vi "setSetpoints.vi"(0 "Interface in":T2, 5 "Setpoint":T1, 7 "Value":sgl, 11 "error in":errorcluster) -> (4 "Interface out":T2, 15 "error out":errorcluster)   [LabVIEW 2017, in "AFE_interface.lvlib"]
uses:
  AFE_interface.lvlib
  InterfaceRef.ctl
  <instrlib>/_niInstr/Instruction Framework/v1/Host/Instruction Target/niInstr Instruction Target v1 Host.lvclass
  <instrlib>/_niInstr/Instruction Framework/v1/Host/Instruction Framework Context/niInstr Instruction Framework Context v1 Host.lvclass
  Setpoints.ctl
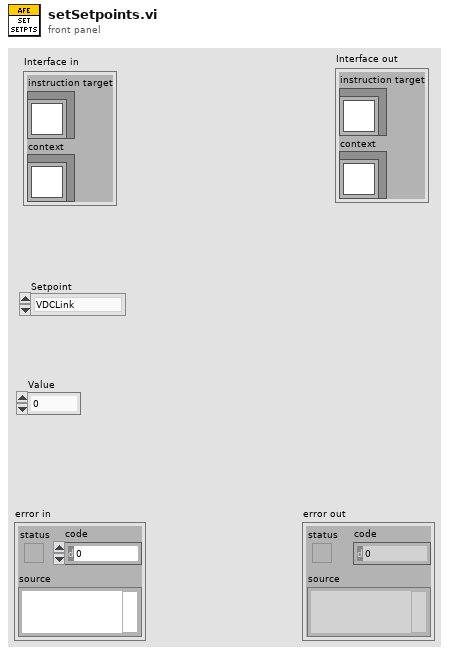
[diagram p1: front panel]
types:
  T1 = typedef "AFE_interface.lvlib/Setpoints.ctl" = enum16{"VDCLink", "Q", "Powerfactor"}
  T2 = typedef "AFE_interface.lvlib/InterfaceRef.ctl" = cluster{"instruction target":refnum<class "niInstr Instruction Target v1 Host.lvclass">, "context":refnum<class "niInstr Instruction Framework Context v1 Host.lvclass">}
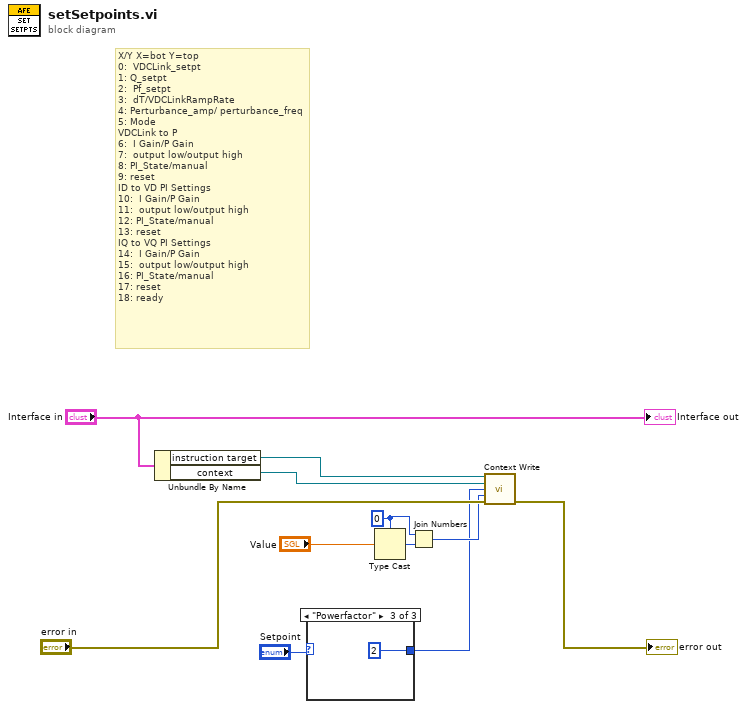
[diagram p0: block diagram]
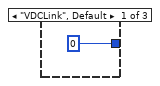
[diagram p2: hidden frame]
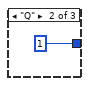
[diagram p3: hidden frame]
diagram:
  w6 = u32 0
  # "X/Y X=bot Y=top\n0:  VDCLink_setpt\n1: Q_setpt\n2:  Pf_setpt\n3:  dT/VDCLinkRampRate\n4: Perturbance_amp/ perturbance_freq\n5: Mode\nVDCLink to P\n6:  I Gain/P Gain\n7:  output low/output high\n8: PI_State/manual\n9: reset\nID to VD PI Settings \n10:  I Gain/P Gain\n11:  output low/output high\n12: PI_State/manual\n13: reset\nIQ to VQ PI Settings\n14:  I Gain/P Gain\n15:  output low/output high\n16: PI_State/manual\n17: reset\n18: ready"
  n1 = Unbundle By Name("Interface in") -> ("instruction target"=w10:refnum<class "niInstr Instruction Target v1 Host.lvclass">, "context"=w9:refnum<class "niInstr Instruction Framework Context v1 Host.lvclass">)
  n2 = case shown="\"Powerfactor\"" "Setpoint" {
    tunnel: [u64 0 ("address") u64 1 ("address") u64 2 ("address")] -> w1
    frame "VDCLink", Default {
    }
    frame "Q" {
    }
    frame "Powerfactor" {
    }
  }
  n3 = Type Cast(type=w6, x="Value") -> (*(type *) &x=w5:u32)
  n4 = Join Numbers(hi=w6, lo=w5) -> ((hi.lo)=w4:u64)
  n5 = call <instrlib>:"Context Write.vi"("instruction target in"=w10, "context in"=w9, "address"=w1, "data"=w4, "error in"="error in") -> ("error out"=→"error out":errorcluster)  [unwired: 8 in, 2 out]
  "Interface out" <- "Interface in"
